vi "SetFormatter.vi"(8 "error in (no error)":errorcluster, 10 "Formatter in":refnum<class "Formatter.lvclass">, 11 "Handler in":refnum<class "Handler.lvclass">) -> (0 "error out":errorcluster, 2 "Formatter out":refnum<class "Formatter.lvclass">, 3 "Handler out":refnum<class "Handler.lvclass">)   [LabVIEW 2022 SP3, in "Logger.lvlib" / "Handler.lvclass"]
uses:
  Handler.lvclass
  Handler.lvclass/Handler.ctl
  Formatter/Formatter.lvclass
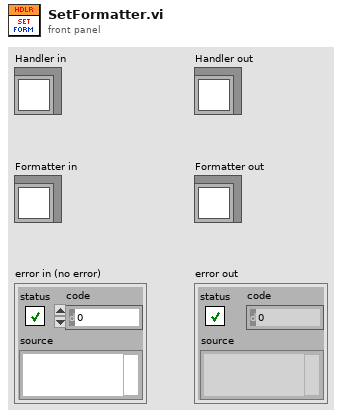
[diagram p1: front panel]
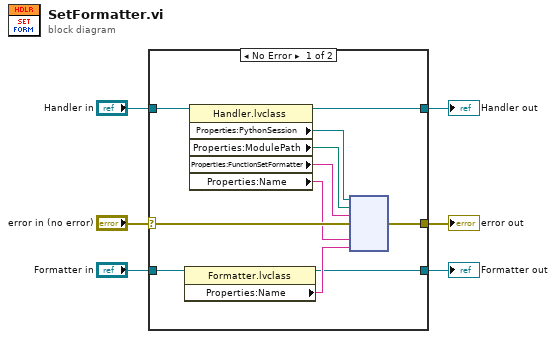
[diagram p0: block diagram]
diagram:
  n1 = case shown="No Error" "error in (no error)" {
    selector: "error in (no error)" -> [w16 w19]
    tunnel: [w15 w19] -> w5
    tunnel: [w7 w18] -> w1
    tunnel: "Handler in" -> [w17 w18]
    tunnel: "Formatter in" -> [w11 _]
    tunnel: [w9 _] -> w3
    frame No Error {
      n2 = property class="Formatter.lvclass"(reference=w11) -> (reference out=w9:refnum<class "Formatter.lvclass">, "Properties:Name"=w10:string)  [unwired: 1 in, 1 out]
      n3 = property class="Handler.lvclass"(reference=w17) -> (reference out=w7:refnum<class "Handler.lvclass">, "Properties:PythonSession"=w14:refnum<k35>, "Properties:ModulePath"=w12:path, "Properties:FunctionSetFormatter"=w13:string, "Properties:Name"=w8:string)  [unwired: 1 in, 1 out]
      n4 = node(w14, w12, w13, w16, w8, w10) -> (w15:errorcluster)  [unwired: 4 in, 3 out]
    }
    frame Error {
    }
  }
  "error out" <- w5
  "Handler out" <- w1
  "Formatter out" <- w3
